vi "createCommand.vi"(8 "error in (no error)":errorcluster, 10 "Command":T1, 11 "CommandFactory in":refnum<class "CommandFactory.lvclass">) -> (0 "error out":errorcluster, 2 "command":refnum<class "Command.lvclass">, 3 "CommandFactory out":refnum<class "CommandFactory.lvclass">)   [LabVIEW 2015, in "CommandFactory.lvclass"]
uses:
  CommandFactory.lvclass
  Command/Command.lvclass
  Typedefs/CommandSelector.ctl
  Commands/Start/Start.lvclass
  Commands/Enable/Enable.lvclass
  Commands/Disable/Disable.lvclass
  Commands/StandBy/Standby.lvclass
  Commands/Exit/Shutdown.lvclass
  Typedefs/FAMTTypedefs.lvlib
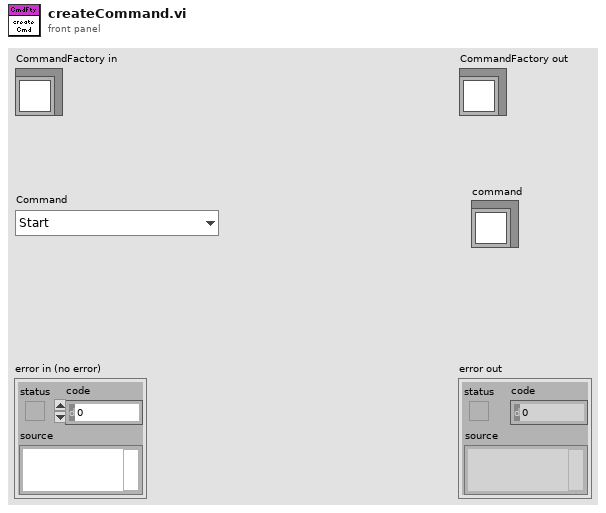
[diagram p1: front panel]
types:
  T1 = typedef "FAMTTypedefs.lvlib/CommandSelector.ctl" = enum16{"Start", "Enable", "Disable", "Standby", "Shutdown"}
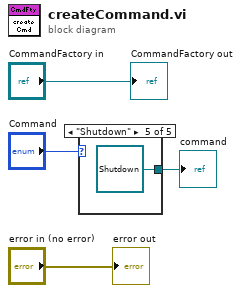
[diagram p0: block diagram]
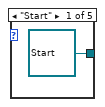
[diagram p2: hidden frame]
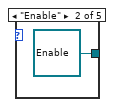
[diagram p3: hidden frame]
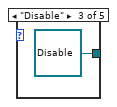
[diagram p4: hidden frame]
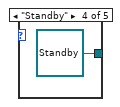
[diagram p5: hidden frame]
diagram:
  n1 = case shown="\"Shutdown\"" "Command" {
    tunnel: [refnum<class "Start.lvclass"> refnum ("Start.lvclass") refnum<class "Enable.lvclass"> refnum ("Enable.lvclass") refnum<class "Disable.lvclass"> refnum ("Disable.lvclass") refnum<class "Standby.lvclass"> refnum ("Standby.lvclass") refnum<class "Shutdown.lvclass"> refnum ("Shutdown.lvclass")] -> w2
    frame "Start" {
    }
    frame "Enable" {
    }
    frame "Disable" {
    }
    frame "Standby" {
    }
    frame "Shutdown" {
    }
  }
  "command" <- w2
  "error out" <- "error in (no error)"
  "CommandFactory out" <- "CommandFactory in"
